vi "60 Hz - ELVIS 2-Level 3-Leg, 3-Phase Inverter Co-simulation v18.vi"() -> ()   [LabVIEW 2012]
uses:
  <vilib>/Simulation/Scripting/Companion Diagram/SimConfigNode/SimParams.ctl
  <vilib>/Simulation/Scripting/Companion Diagram/SimConfigNode/_simSolvers.ctl
  <vilib>/Simulation/Implementation/Shared/SIMSCR Execution Mode.ctl
  <vilib>/Simulation/Param Hierarchy/Typedefs/SIMPH Param Control Actions.ctl
  <vilib>/Simulation/Scripting/Editor Utilities/SIM subVI tag data.ctl
  <vilib>/Simulation/Scripting/Editor Utilities/SIM subVI execution type.ctl
  <vilib>/Simulation/Implementation/Shared/NILVSim_ParamChanged.vi
  <vilib>/Simulation/Utility/Implementation/SIM Halt.vi
  <vilib>/Simulation/Utility/Implementation/NILVSim Indexer (Imp).llb/SIM Index by Time (Waveform).vi
  <vilib>/Simulation/Implementation/Shared/SIM Fire Discrete SubVI.vi
  <vilib>/Simulation/SignalDisplay/Implementation/NILVSim Time Waveform.llb/SIM Time Waveform (vector).vi
  <vilib>/Simulation/Implementation/Shared/NILVSim_Manager.vi
  <vilib>/Simulation/Implementation/Shared/NILVSim_FinalizeModel.vi
  <vilib>/Simulation/Utility/Implementation/NILVSim Indexer (Imp).llb/NILVSim Index by Time Core (Waveform).vi
  <vilib>/Simulation/Implementation/Shared/SIM Interpolate.llb/SIM Interpolate (Waveform).vi
  <vilib>/Simulation/Implementation/Shared/SIM Fire Discrete SubVI (Core).vi
  <vilib>/Simulation/Implementation/Shared/SIM Interpolate.llb/SIM Interpolate (array).vi
  <vilib>/Simulation/Implementation/Shared/SIM Unbundle Sim Info.vi
  <vilib>/Utility/error.llb/Clear Errors.vi
  <vilib>/Simulation/Implementation/Shared/NILVSim_GetModelError.vi
  <vilib>/Simulation/Implementation/Shared/SIM Bundle Sim Info.vi
  <vilib>/Simulation/Implementation/Shared/SIMSH Read Queue.vi
  <vilib>/Simulation/Implementation/Shared/NILVSim_Initialize.vi
  <vilib>/Simulation/Utility/Implementation/NILVSim Get Time and IsAcceptedStep.vi
  IP Cores/IP Cores - LabVIEW FPGA/Control & Signal Gen/FPGA FXPT TriangleGen with Mod Index (use inside SCTL).vi
  IP Cores/IP Cores - LabVIEW FPGA/Control & Signal Gen/FPGA Rising edge delay (Use inside SCTL).vi
  <vilib>/Simulation/Scripting/Companion Diagram/SimConfigNode/SimDog.xnode
  <vilib>/Simulation/Implementation/XNodeFramework/SimXNode/SimX.xnode
  <vilib>/rvi/FXPMathLib/basic elements/FxpDiscreteDelay/XNode/nifxpmath_DiscreteDelay.xnode
  <vilib>/Simulation/EMI/Plugins/Multisim Design/MultisimEMICtrl.dll
  <vilib>/Simulation/Implementation/Shared/NI_SIM_Implementation.lvlib
panel:
  out "Chart 3":waveform(dbl)[](graph)
  out "Chart 1":waveform(dbl)[](graph)
  out "Vgrid_ab":fxp<+/-,18,11>
  out "Vgrid_bc":fxp<+/-,18,11>
  in  "PLL PI gains":T1={"proportional gain (Kp)"=0.1201171875, "integral gain (Ki)"=16.0}
  in  "PLL anti-windup\ngain (Ka)":fxp<+,16,9>=16.0
  out "PLL Frequency (Hz)":fxp<+,18,8>
  out "PLL_Sine_B":fxp<+/-,18,2> format="%#.6g"
  out "PLL_Sine_C":fxp<+/-,18,2>
  out "PLL_Sine_A":fxp<+/-,18,2>
  in  "B Shift (deg)":u16
  in  "A Shift (deg)":u16=240
  in  "C Shift (deg)":u16=120
  out "Chart 2":waveform(dbl)[](graph)
  out "Carrier Freq. \n(=fc(Hz)*4/50e6)":dbl=0.00039999978616833687 format="%.2f"
  in  "Deadtime (iterations)":i16=1
  in  "Enable\nDAQ":bool
  in  "Halt?":bool
  in  "Discrete Step Size (s)":dbl=4.63e-06
  in  "Mod Index (0..2)":dbl=1.0
  in  "fc, PWM carrier \nfrequency (Hz)":dbl=4000.0
  out "phA_U":bool
  out "phB_U":bool
  out "phC_U":bool
  out "phA_L":bool
  out "phB_L":bool
  out "phC_L":bool
  out "swA_U":bool
  out "swB_U":bool
  out "swC_U":bool
  out "swA_L":bool
  out "swB_L":bool
  out "swC_L":bool
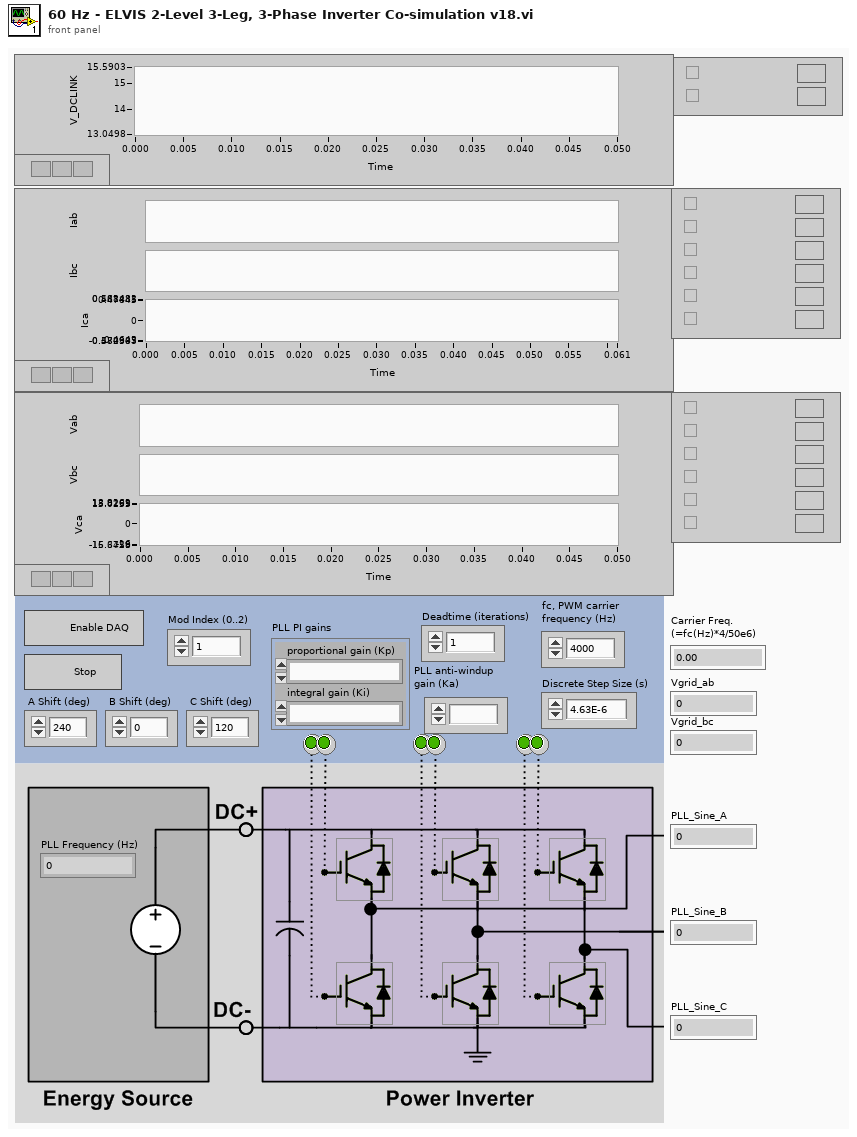
[diagram p1: front panel]
types:
  T1 = cluster{"proportional gain (Kp)":fxp<+,16,6>, "integral gain (Ki)":fxp<+,16,9>}
  T2 = enum16{"Runge-Kutta 1 (Euler)", "Runge-Kutta 2", "Runge-Kutta 3", "Runge-Kutta 4", "Runge-Kutta 23 (variable)", "Runge-Kutta 45 (variable)", "BDF (variable)", "Adams-Moulton (variable)", "Rosenbrock (variable)", "Discrete States Only"}
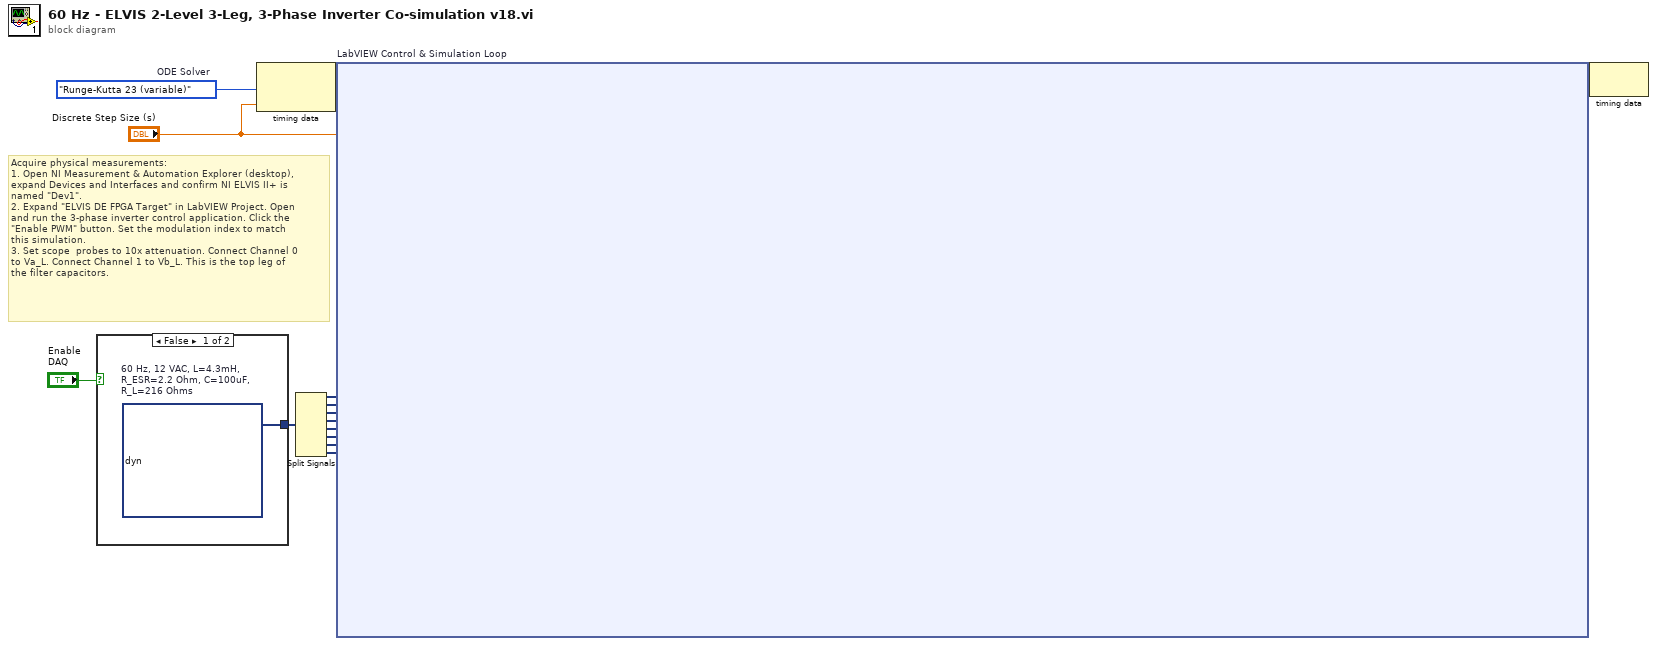
[diagram p0: block diagram]
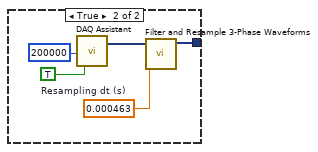
[diagram p2: hidden frame]
diagram:
  w1 = T2."Runge-Kutta 23 (variable)"  # ODE Solver
  # "Acquire physical measurements:\n1. Open NI Measurement & Automation Explorer (desktop),\nexpand Devices and Interfaces and confirm NI ELVIS II+ is \nnamed \"Dev1\".\n2. Expand \"ELVIS DE FPGA Target\" in LabVIEW Project. Open \nand run the 3-phase inverter control application. Click the\n\"Enable PWM\" button. Set the modulation index to match\nthis simulation.\n3. Set scope  probes to 10x attenuation. Connect Channel 0\nto Va_L. Connect Channel 1 to Vb_L. This is the top leg of\nthe filter capacitors."
  n1 = case shown="False" "Enable\nDAQ" {
    tunnel: [w15 w17] -> w3
    frame False {
      w15 = dynamicdata [{"t0"=timestamp(0 s since 1904-01-01), "dt"=0.000463, "Y"=array[11988 elements], "attributes"=variant("NI_ChannelName"=variant(string "Vab_grid"))}, {"t0"=timestamp(0 s since 1904-01-01), "dt"=0.000463, "Y"=array[11988 elements], "attributes"=variant("NI_ChannelName"=variant(string "V_DCLINK"))}, {"t0"=timestamp(0 s since 1904-01-01), "dt"=0.000463, "Y"=array[11988 elements], "attributes"=variant("NI_ChannelName"=variant(string "Vab_L"))}, {"t0"=timestamp(0 s since 1904-01-01), "dt"=0.000463, "Y"=array[11988 elements], "attributes"=variant("NI_ChannelName"=variant(string "Vbc_L"))}, {"t0"=timestamp(0 s since 1904-01-01), "dt"=0.000463, "Y"=array[11988 elements], "attributes"=variant("NI_ChannelName"=variant(string "Vca_L"))}, {"t0"=timestamp(0 s since 1904-01-01), "dt"=0.000463, "Y"=array[11988 elements], "attributes"=variant("NI_ChannelName"=variant(string "Iab_i"))}, {"t0"=timestamp(0 s since 1904-01-01), "dt"=0.000463, "Y"=array[11988 elements], "attributes"=variant("NI_ChannelName"=variant(string "Ibc_i"))}, {"t0"=timestamp(0 s since 1904-01-01), "dt"=0.000463, "Y"=array[11988 elements], "attributes"=variant("NI_ChannelName"=variant(string "Ica_i"))}, {"t0"=timestamp(0 s since 1904-01-01), "dt"=0.000463, "Y"=array[11988 elements], "attributes"=variant("NI_ChannelName"=variant(string "Vab_i"))}, {"t0"=timestamp(0 s since 1904-01-01), "dt"=0.000463, "Y"=array[11988 elements], "attributes"=variant("NI_ChannelName"=variant(string "Vbc_i"))}, {"t0"=timestamp(0 s since 1904-01-01), "dt"=0.000463, "Y"=array[11988 elements], "attributes"=variant("NI_ChannelName"=variant(string "Vca_i"))}, {"t0"=timestamp(0 s since 1904-01-01), "dt"=0.000463, "Y"=array[11988 elements], "attributes"=variant("NI_ChannelName"=variant(string "Va_L"))}, {"t0"=timestamp(0 s since 1904-01-01), "dt"=0.000463, "Y"=array[11988 elements], "attributes"=variant("NI_ChannelName"=variant(string "Vb_L"))}, {"t0"=timestamp(0 s since 1904-01-01), "dt"=0.000463, "Y"=array[11988 elements], "attributes"=variant("NI_ChannelName"=variant(string "Vc_L"))}]  # 60 Hz, 12 VAC, L=4.3mH, R_ESR=2.2 Ohm, C=100uF, R_L=216 Ohms
    }
    frame True {
      w16 = 0.000463  # Resampling dt (s)
      n2 = call "DAQ Assistant"("number of samples"=200000, "stop (F)"=TRUE) -> ("data"=w18:dynamicdata)  [unwired: 14 in, 3 out]
      n3 = call "Filter and Resample 3-Phase Waveforms.vi"("Resampling dt (s)"=w16, "Dynamic Data In"=w18) -> ("Dynamic Data Out"=w17:dynamicdata)  [unwired: 8 in, 1 out]
    }
  }
  n4 = node-c288(w1, "Discrete Step Size (s)") -> (w14:variant)
  n5 = Split Signals(w3) -> (w11:dynamicdata, w4:dynamicdata, w10:dynamicdata, w9:dynamicdata, w8:dynamicdata, w7:dynamicdata, w6:dynamicdata, w5:dynamicdata)  [unwired: 8 in]
  n6 = node-c254 "LabVIEW Control & Simulation Loop"(w14, w11, w10, w9, w8, w7, w6, w5, w4, "Discrete Step Size (s)") -> (w13:variant)
  n7 = node-c288(w13) -> ()  [unwired: 1 out]
